vi "S2C_5190CR_Poly_TestBed.vi"() -> ()   [LabVIEW 2015]
uses:
  S2C_5190CR_Poly_Initialize.vi
  S2C_5190CR_Poly_MeasureCurrent.vi
  S2C_5190CR_Poly_MeasurePower.vi
  S2C_5190CR_Poly_MeasureVoltage.vi
  S2C_5190CR_Poly_SetOutput.vi
panel:
  out "Error Out":errorcluster
  in  "Error In":errorcluster
  out "Response":T1
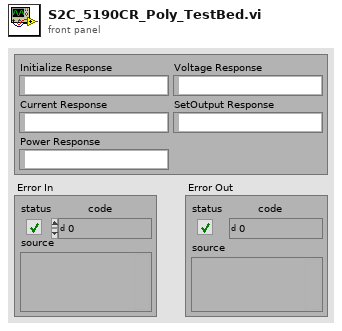
[diagram p1: front panel]
types:
  T1 = cluster{"Initialize Response":string, "Current Response":string, "Power Response":string, "Voltage Response":string, "SetOutput Response":string}
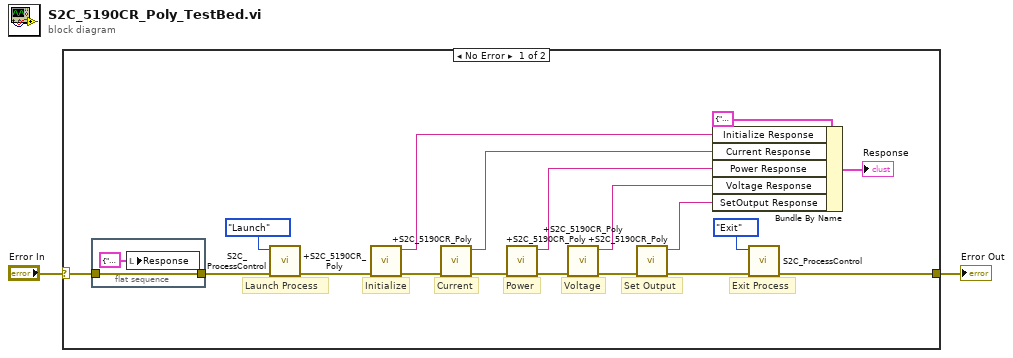
[diagram p0: block diagram]
diagram:
  n1 = case shown="No Error" "Error In" {
    selector: "Error In" -> [w17 w23]
    tunnel: [w18 w23] -> w1
    frame No Error {
      # "Set Output"
      # "Voltage"
      # "Power"
      # "Current"
      # "Initialize"
      # "Exit Process"
      # "Launch Process"
      n2 = flat-sequence {
        tunnel: w17 -> [w22]
        tunnel: [w22] -> w16
        frame #0 {
          n3 = local write "Response"(T1 {"Initialize Response"="", "Current Response"="", "Power Response"="", "Voltage Response"="", "SetOutput Response"=""} ("Response")) -> ()
        }
      }
      n4 = call "S2C_ProcessControl.vi"("Error In"=w16, "Action"=enum16{"Launch", "Exit"}."Launch") -> ("Error Out"=w15:errorcluster)  [unwired: 9 in]
      n5 = call-poly "+S2C_5190CR_Poly.vi"("Error In"=w15) -> ("Error Out"=w14:errorcluster, "Response"=w13:string)  [unwired: 9 in]
      n6 = call-poly "+S2C_5190CR_Poly.vi"("Error In"=w14) -> ("Error Out"=w5:errorcluster, "Response"=w12:string)  [unwired: 9 in]
      n7 = call-poly "+S2C_5190CR_Poly.vi"("Error In"=w5) -> ("Error Out"=w4:errorcluster, "Response"=w11:string)  [unwired: 9 in]
      n8 = call-poly "+S2C_5190CR_Poly.vi"("Error In"=w4) -> ("Error Out"=w3:errorcluster, "Response"=w10:string)  [unwired: 9 in]
      n9 = call-poly "+S2C_5190CR_Poly.vi"("Error In"=w3) -> ("Error Out"=w8:errorcluster, "Response"=w9:string)  [unwired: 9 in]
      n10 = Bundle By Name(cluster=T1 {"Initialize Response"="", "Current Response"="", "Power Response"="", "Voltage Response"="", "SetOutput Response"=""} ("Response"), "Initialize Response"=w13, "Current Response"=w12, "Power Response"=w11, "Voltage Response"=w10, "SetOutput Response"=w9) -> (→"Response":T1)
      n11 = call "S2C_ProcessControl.vi"("Error In"=w8, "Action"=enum16{"Launch", "Exit"}."Exit") -> ("Error Out"=w18:errorcluster)  [unwired: 9 in]
    }
    frame Error {
    }
  }
  "Error Out" <- w1
